vi "Init.vi"(8 "error in (no error)":errorcluster, 11 "Communication Channel in":refnum<class "Communication Channel.lvclass">) -> (0 "error out":errorcluster, 3 "Communication Channel out":refnum<class "Communication Channel.lvclass">)   [LabVIEW 2018, in "Communication Channel.lvclass"]
uses:
  Communication Channel.lvclass
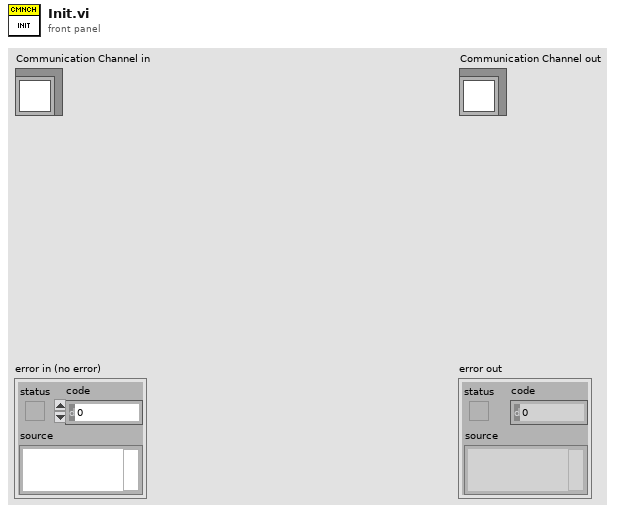
[diagram p1: front panel]
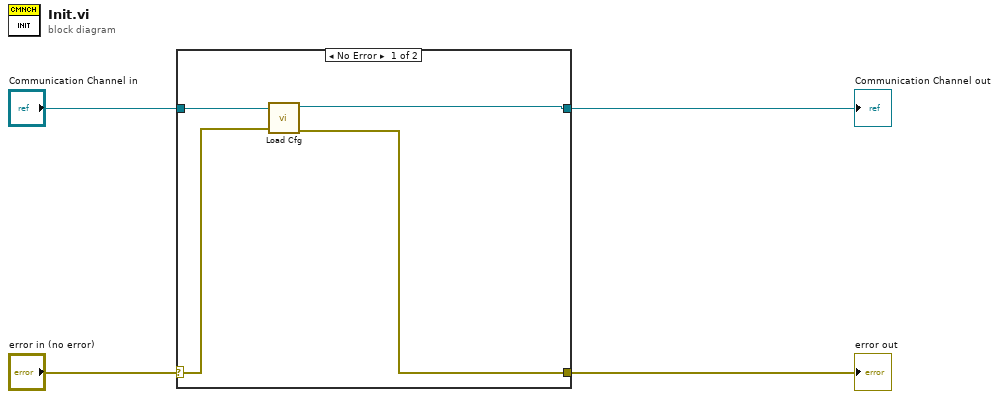
[diagram p0: block diagram]
diagram:
  n1 = case shown="No Error" "error in (no error)" {
    selector: "error in (no error)" -> [w7 w10]
    tunnel: [w5 w10] -> w3
    tunnel: [w6 w9] -> w1
    tunnel: "Communication Channel in" -> [w8 w9]
    frame No Error {
      n2 = call-dynamic "Load Cfg.vi"("error in (no error)"=w7, "Communication Channel in"=w8) -> ("error out"=w5:errorcluster, "Communication Channel out"=w6:refnum<class "Communication Channel.lvclass">)  [unwired: 8 in]
    }
    frame Error {
    }
  }
  "error out" <- w3
  "Communication Channel out" <- w1
